vi "AMI_LevelMeter 2.vi"(6 "address string":string="1") -> (2 "level":dbl)   [LabVIEW 2019]
panel:
  out "data":string
  out "# of additional attempts":i32
  out "error out":errorcluster
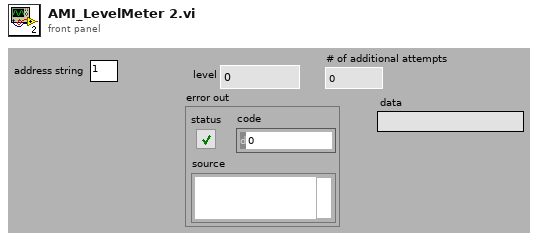
[diagram p1: front panel]
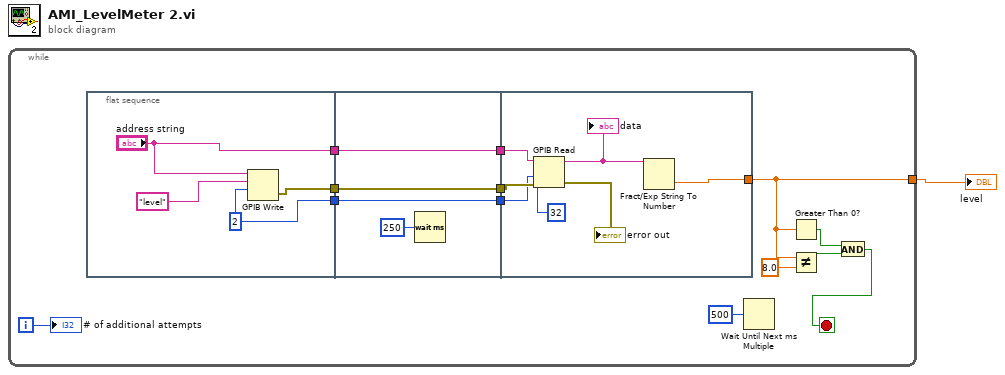
[diagram p0: block diagram]
diagram:
  n1 = while {
    tunnel: [w6] -> w1
    i -> [w7]
    stop <- w2 stop-if-true
    n2 = flat-sequence {
      tunnel: [w15] -> w14
      tunnel: ["address string"] -> w13
      tunnel: [w17] -> w12
      tunnel: [w22] -> w11
      tunnel: [w21] -> w10
      tunnel: [w20] -> w9
      tunnel: w14 -> [w22]
      tunnel: w13 -> [w21]
      tunnel: w12 -> [w20]
      tunnel: w11 -> [w29]
      tunnel: w10 -> [w28]
      tunnel: w9 -> [w27]
      tunnel: [w23] -> w6
      frame #0 {
        w17 = i16 2 ("mode (0)")
        n3 = GPIB Write(0:"address string", 1:"level" ("data"), 2:w17) -> (6:w15:errorcluster)  [unwired: 2 in, 1 out]
      }
      frame #1 {
        n4 = Wait (ms)(milliseconds to wait=u32 250) -> ()  [unwired: 1 out]
      }
      frame #2 {
        n5 = GPIB Read(0:w28, 1:32 ("byte count"), 2:w27, 3:w29) -> (5:w26:string, 7:→"error out":errorcluster)  [unwired: 1 in, 1 out]
        "data" <- w26
        n6 = Fract/Exp String To Number(string=w26) -> (number=w23:dbl)  [unwired: 3 in, 1 out]
      }
    }
    n7 = Wait Until Next ms Multiple(millisecond multiple=u32 500) -> ()  [unwired: 1 out]
    n8 = Greater Than 0?(x=w6) -> (x > 0?=w4:bool)
    n9 = Not Equal?(x=w6, y=8.0) -> (x != y?=w3:bool)
    n10 = And(x=w4, y=w3) -> (x .and. y?=w2:bool)
    "# of additional attempts" <- w7
  }
  "level" <- w1
